vi "Task Awaiter.vi"(8 "error in (no error)":errorcluster, 10 "Timeout":i32=-1, 11 "Task":refnum<k24>) -> (0 "error out":errorcluster, 2 "Timeout":bool, 3 "Task":refnum<k24>)   [LabVIEW 2020, in "WebView2.lvlib" / "WebView2 Control.lvclass"]
uses:
  WebView2 Control.lvclass
  WebView2 Control.lvclass/WebView2 Control.ctl
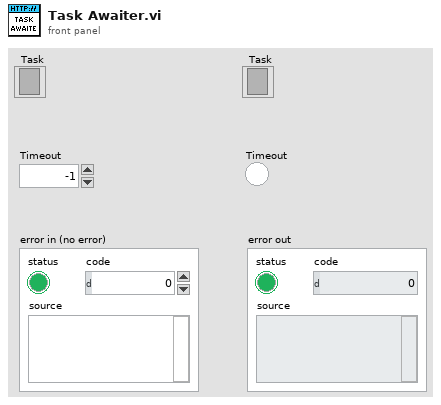
[diagram p1: front panel]
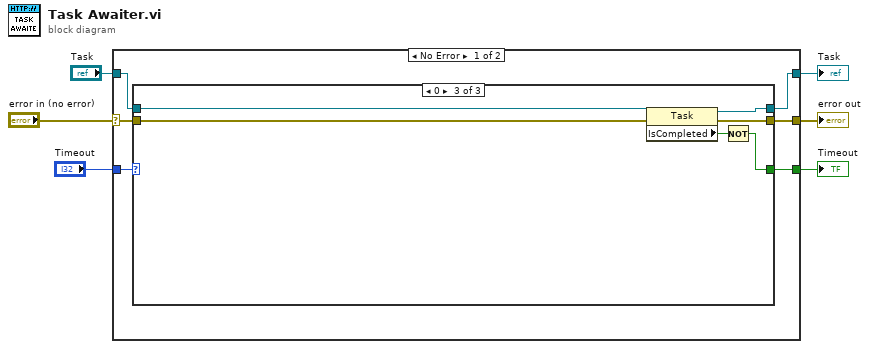
[diagram p0: block diagram]
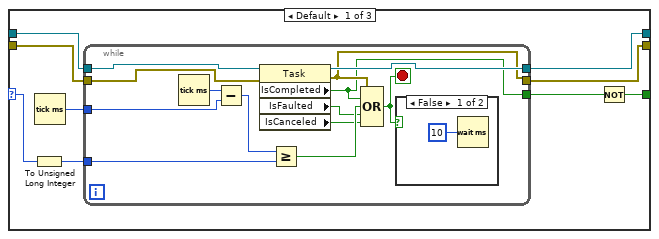
[diagram p2: hidden frame]
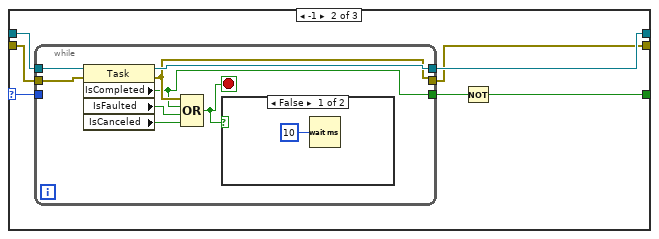
[diagram p4: hidden frame]
diagram:
  n1 = case shown="No Error" "error in (no error)" {
    selector: "error in (no error)" -> [w11 w59]
    tunnel: "Task" -> [w12 w58]
    tunnel: "Timeout" -> [w10 _]
    tunnel: [w9 w59] -> w3
    tunnel: [w8 w58] -> w2
    tunnel: [w7 _] -> w1
    frame No Error {
      n2 = case shown="0" w10 {
        selector: w10 -> [w18 w39 _]
        tunnel: w12 -> [w21 w42 w57]
        tunnel: w11 -> [w20 w41 w56]
        tunnel: [w19 w40 w55] -> w8
        tunnel: [w17 w38 w52] -> w9
        tunnel: [w16 w36 w53] -> w7
        frame Default {
          n3 = To Unsigned Long Integer(number=w18) -> (unsigned 32bit integer=w13:u32)
          n4 = Tick Count (ms)() -> (millisecond timer value=w15:u32)
          n5 = while {
            tunnel: w21 -> [w34]
            tunnel: w20 -> [w33]
            tunnel: [w32] -> w19
            tunnel: w15 -> [w30]
            tunnel: w13 -> [w28]
            tunnel: [w26] -> w17
            tunnel: [w25] -> w14
            stop <- w22 stop-if-true
            n6 = Tick Count (ms)() -> (millisecond timer value=w31:u32)
            n7 = Subtract(x=w31, y=w30) -> (x-y=w29:u32)
            n8 = property class="Task"(reference=w34, error in=w33) -> (reference out=w32:refnum<k24>, error out=w26:errorcluster, "IsCompleted"=w25:bool, "IsFaulted"=w24:bool, "IsCanceled"=w23:bool)
            n9 = Greater Or Equal?(x=w29, y=w28) -> (x >= y?=w27:bool)
            n10 = Compound Arithmetic op=OR(w26, w25, w27, w24, w23) -> (w22:bool)
            n11 = case shown="False" w22 {
              frame False {
                n12 = Wait (ms)(milliseconds to wait=u32 10) -> ()  [unwired: 1 out]
              }
              frame True {
              }
            }
          }
          n13 = Not(x=w14) -> (.not. x?=w16:bool)
        }
        frame -1 {
          n14 = while {
            tunnel: w42 -> [w50]
            tunnel: w41 -> [w49]
            tunnel: [w48] -> w40
            tunnel: w39 -> [_]
            tunnel: [w47] -> w38
            tunnel: [w46] -> w37
            stop <- w43 stop-if-true
            n15 = property class="Task"(reference=w50, error in=w49) -> (reference out=w48:refnum<k24>, error out=w47:errorcluster, "IsCompleted"=w46:bool, "IsFaulted"=w45:bool, "IsCanceled"=w44:bool)
            n16 = Compound Arithmetic op=OR(w47, w46, w45, w44) -> (w43:bool)
            n17 = case shown="False" w43 {
              frame False {
                n18 = Wait (ms)(milliseconds to wait=u32 10) -> ()  [unwired: 1 out]
              }
              frame True {
              }
            }
          }
          n19 = Not(x=w37) -> (.not. x?=w36:bool)
        }
        frame 0 {
          n20 = property class="Task"(reference=w57, error in=w56) -> (reference out=w55:refnum<k24>, error out=w52:errorcluster, "IsCompleted"=w54:bool)
          n21 = Not(x=w54) -> (.not. x?=w53:bool)
        }
      }
    }
    frame Error {
    }
  }
  "error out" <- w3
  "Task" <- w2
  "Timeout" <- w1
